vi "CCD_Initialization.vi"(0 "CCD GPIB Address":i16=1 min=1 max=1, 1 "milliseconds to wait":u32=1000, 2 "Setup String":string="LDu,0,256,8;SDu,0,1024,1024;CL4;OMrm;SRon", 3 "error in":errorcluster, 4 "Starting Action":T1(ring)=enum."Init GPIB") -> (5 "Setup String sent":string="ldu,0,256,16;sdu,0,1024,1024;cl0;omrm;sron", 6 "Poll Byte":i16, 7 "Poll Status":bool[](array[boolean]), 8 "Error (0=No Error)":i16=-1, 9 "error out":errorcluster)   [LabVIEW 2020]
doc: "Resets the CCD camera controller and initializes it with Setup String. The default Setup String is \"ldb,1,16,u,0,225,25,b,1,15;sdu,0,1024,1024;cl0;omrm;sron\". \nError, if no -1, is set as 0 if a serial poll detects an error (bit 15 in status bit set)\n\nSet the CCD Setup String Global variable after the command is complete."
uses:
  Globals and TypeDefs/Type Definitions.llb/3 way Status.ctl
  Globals and TypeDefs/Error Categories.ctt
  Globals and TypeDefs/gStatus.vi
  Globals and TypeDefs/gDetector.vi
panel:
  in  "Case Constant\n(See Context Help)":bool=TRUE
  out "Current Action":T1(ring)=enum."Init GPIB"
  in  "milliseconds to wait in begin":u32=1000
  out "Poll Status 2":bool[](array[boolean])
  out "SRQWait":errorcluster
  out "SRQ Poll":bool[](array[boolean])
  out "SRQ":bool
  out "SetupTime (ms)":u32=3
  out "Poll StatusNo":u16
  out "GPIB Error":u16
  # "Status Byte:\n[0]: Dev.Clear State  \n[1]: Dev.Trig.State    \n[2]: Listener Active   \n[3]: Talker Active      \n[4]: Attn. Asserted    \n[5]: CIC                      \n[6]: Remote State       \n[7]: Lockout State      \n[8]: Oper.Complete\n[9]:   ---\n[10]: ---\n[11]: ---\n[12]: SRQ det.whl CIC\n[13]: EOI or EOS det.\n[14]: Timeout\n[15]: Error detected"
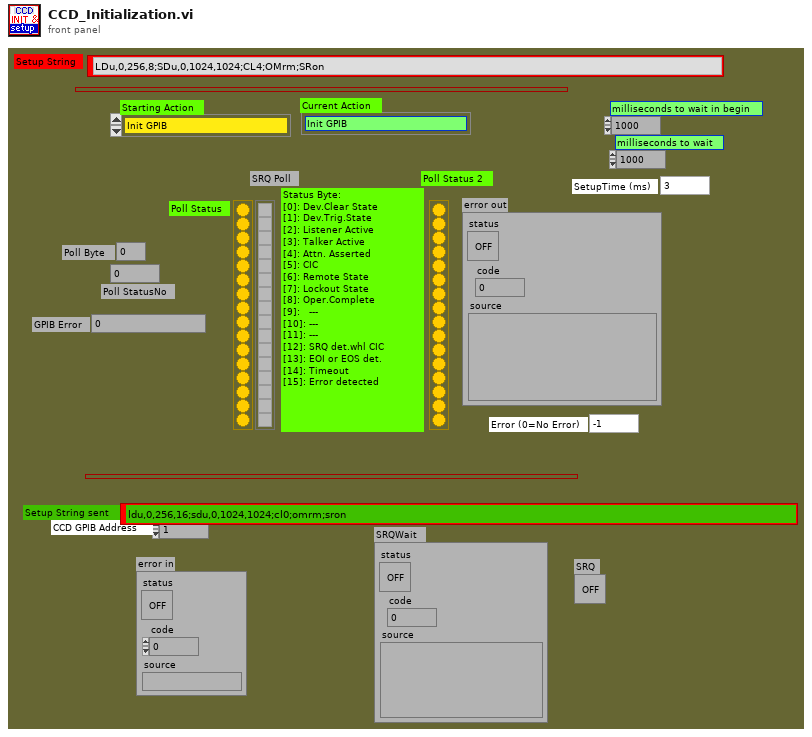
[diagram p1: front panel]
types:
  T1 = enum16{"--Quit--", "Init GPIB", "Poll GPIB", "Wait for SRQ", "Clear CCD Parameters", "New CCD Parameters", "Check CCD Command Error"}
  T2 = enum8{"Initialization Error", "Command Error", "Parameter Error", "Overflow Error", "Time-out Error", "Misc Error", "User cancel"}
  T3 = typedef "Error Categories.ctt" = enum8{"General", "CCD-256x1024", "CCD-1340x400", "InGaAs PDA", "McPherson 2075", "Magnetic Field", "Temperature Control", "Other"}
  T4 = enum16{"Poll CCD GPIB Status", "Check CCD Command Error", "CheckSRQ-Poll"}
  T5 = typedef "3 way Status.ctl" = u8
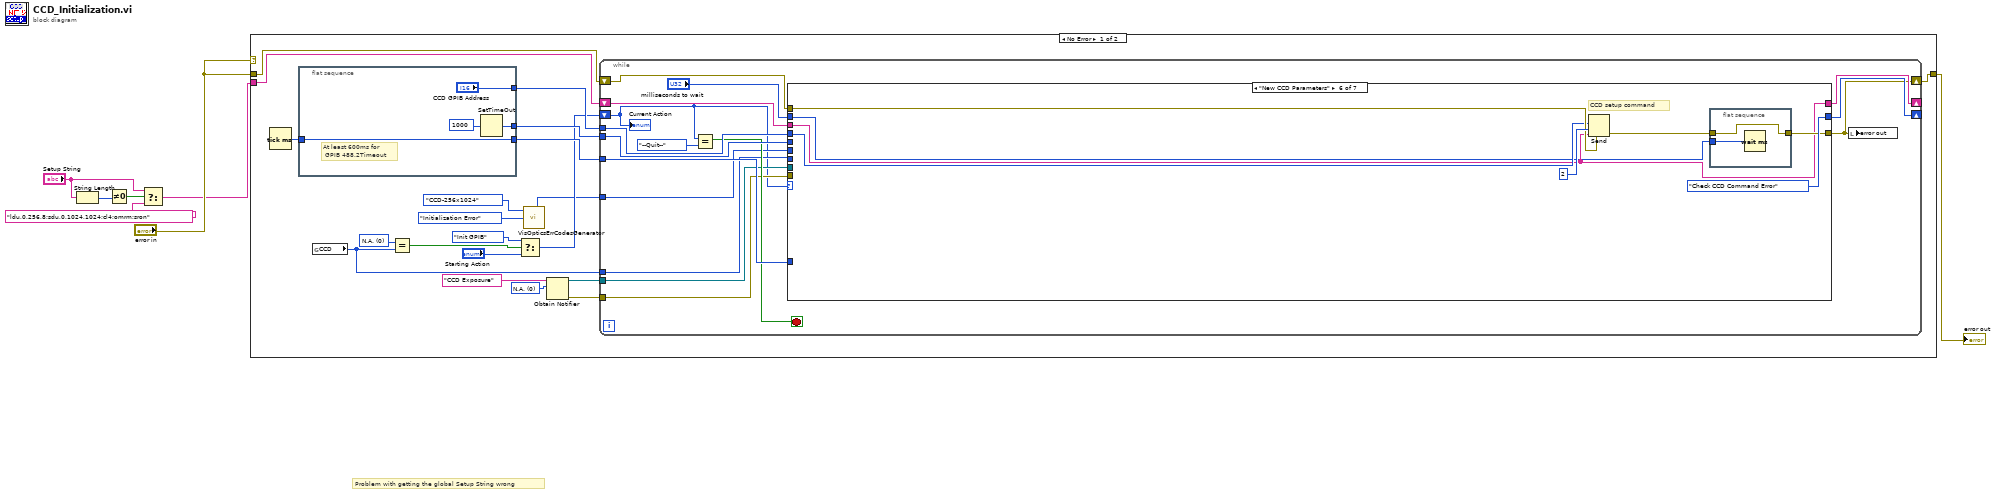
[diagram p0: block diagram]
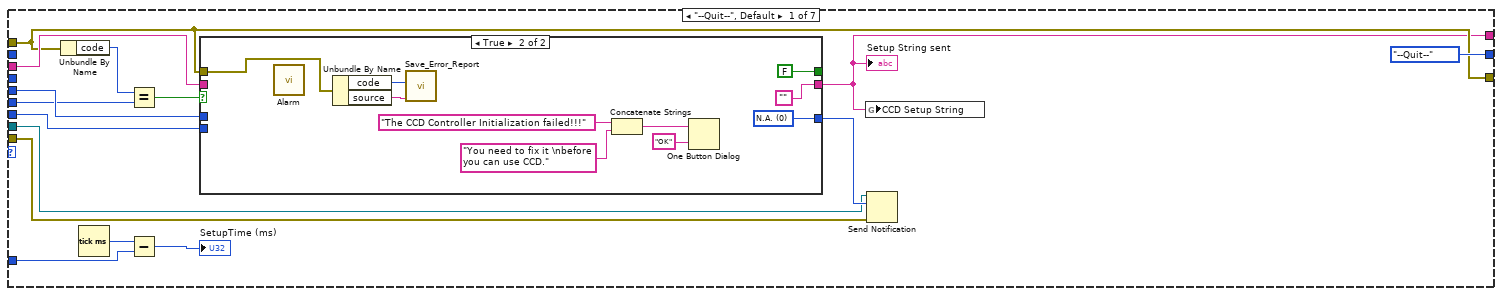
[diagram p2: hidden frame]
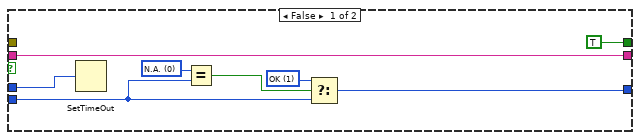
[diagram p3: hidden frame]
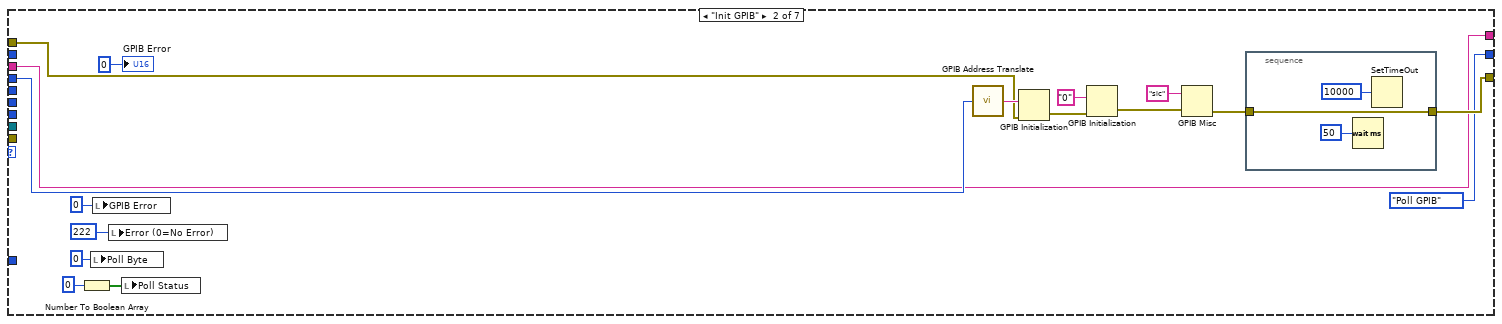
[diagram p4: hidden frame]
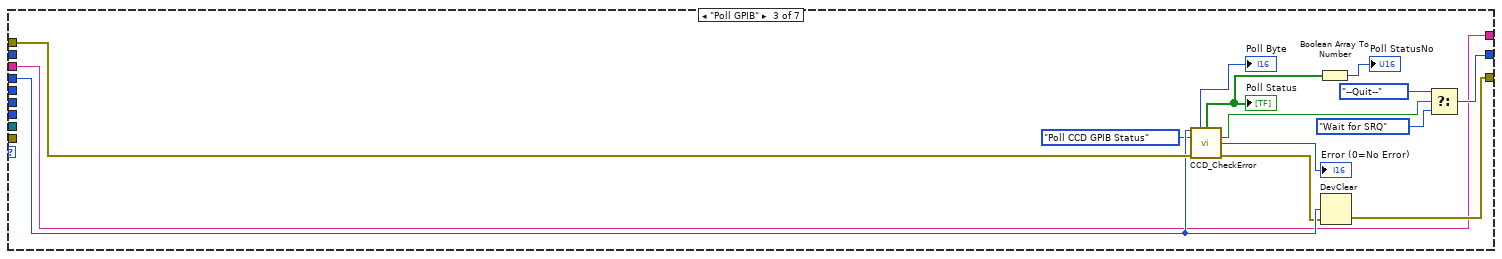
[diagram p5: hidden frame]
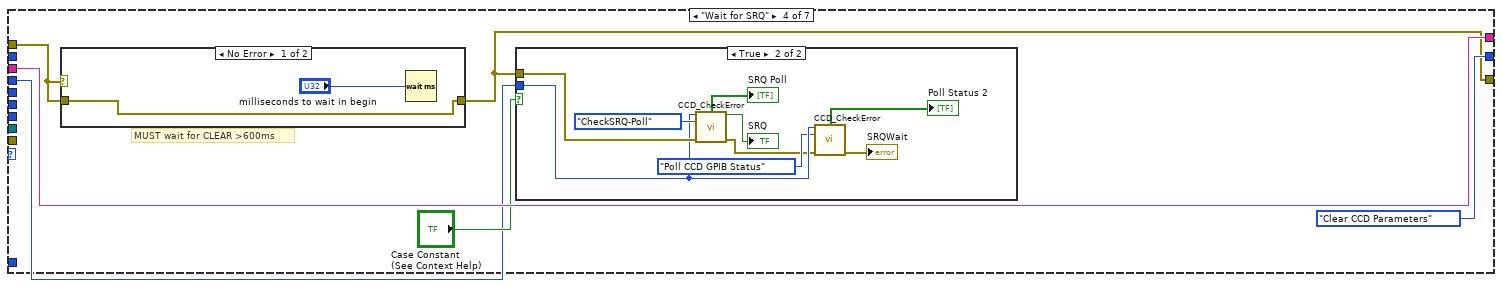
[diagram p6: hidden frame]
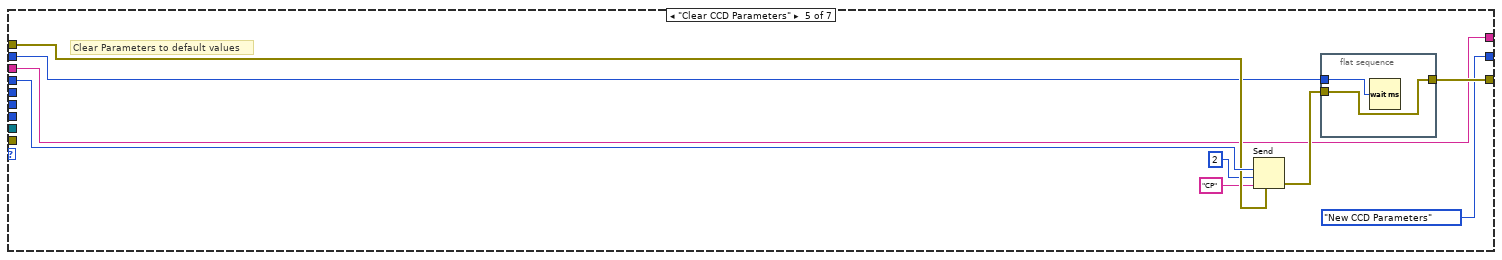
[diagram p9: hidden frame]
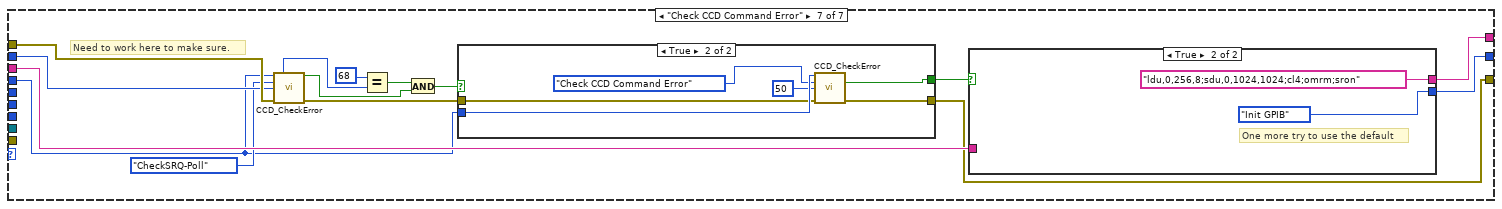
[diagram p10: hidden frame]
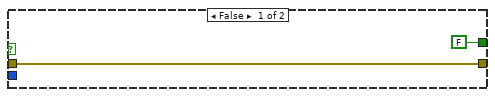
[diagram p11: hidden frame]
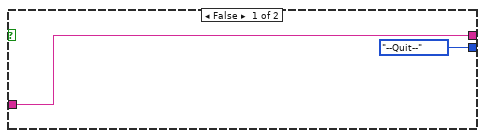
[diagram p12: hidden frame]
diagram:
  # "Problem with getting the global Setup String wrong"
  n1 = String Length(string="Setup String") -> (length=w5:i32)
  n2 = Not Equal To 0?(x=w5) -> (x != 0?=w3:bool)
  n3 = Select(t="Setup String", s=w3, f="ldu,0,256,8;sdu,0,1024,1024;cl4;omrm;sron") -> (s? t:f=w1:string)
  n4 = case shown="No Error" "error in" {
    tunnel: "error in" -> [w27 w181]
    tunnel: [w25 w181] -> w7
    tunnel: w1 -> [w8 _]
    frame No Error {
      w14 = T5 0 items=["N.A.", "OK", "Busy", "Done"] ("Saving")
      w17 = T5 0 items=["N.A.", "OK", "Busy", "Done"] ("y")
      n5 = Tick Count (ms)() -> (millisecond timer value=w23:u32)
      n6 = flat-sequence {
        tunnel: ["CCD GPIB Address"] -> w26
        tunnel: [w30] -> w24
        tunnel: w23 -> [w28]
        tunnel: [w28] -> w22
        frame #0 {
          # "At least 600ms for \n GPIB 488.2Timeout"
          n7 = SetTimeOut(1:1000 ("new timeout (10000)")) -> (0:w30:i32)
        }
      }
      n8 = global read "gStatus.vi" "CCD"() -> (w16:T5)
      n9 = Equal?(x=w17, y=w16) -> (x = y?=w21:bool)
      n10 = Select(t=T1."Init GPIB", s=w21, f="Starting Action") -> (s? t:f=w19:T1)
      n11 = call "VisOpticsErrCodesGenerator.vi"("NHMFL Visible Optics Error Type"=T2."Initialization Error", "NHMFL Visible Optics Error Categories"=Error_Categories.ctt."CCD-256x1024") -> ("User-defined Error Code"=w9:i32)  [unwired: 1 in, 5 out]
      n12 = Obtain Notifier(name (unnamed)="CCD Exposure", notification data type=w14) -> (notifier out=w13:refnum<notifier>, error out=w12:errorcluster)  [unwired: 2 in, 1 out]
      n13 = while {
        shift-right: [w32] -> w25
        shift-left: w27 -> [w47]
        tunnel: w22 -> [w45]
        tunnel: w26 -> [w46]
        tunnel: w24 -> [w44]
        shift-right: [w41] -> _
        shift-left: w19 -> [w33]
        shift-right: [w39] -> _
        shift-left: w8 -> [w40]
        tunnel: w13 -> [w38]
        tunnel: w12 -> [w37]
        tunnel: w16 -> [w34]
        tunnel: w9 -> [w36]
        stop <- w43 stop-if-true
        n14 = Equal?(x=w33, y=T1."--Quit--" ("Starting Action")) -> (x = y?=w43:bool)
        n15 = case shown="\"New CCD Parameters\"" w33 {
          tunnel: w47 -> [w50 w86 w110 w120 w140 w150 w165]
          tunnel: w46 -> [_ w85 w109 w115 w141 w148 w162]
          tunnel: [w50 w83 w103 w117 w137 w146 w154] -> w32
          tunnel: w40 -> [w57 w81 w101 w118 w135 w145 w166]
          tunnel: w45 -> [w62 _ _ _ _ _ _]
          tunnel: w44 -> [w59 _ _ _ _ _ _]
          tunnel: [T1."--Quit--" ("Starting Action") T1."Poll GPIB" ("Starting Action") w114 T1."Clear CCD Parameters" ("Starting Action") T1."New CCD Parameters" ("Starting Action") T1."Check CCD Command Error" ("Starting Action") w168] -> w41
          tunnel: [w49 w81 w101 w118 w135 w145 w167] -> w39
          tunnel: w38 -> [w55 _ _ _ _ _ _]
          tunnel: w37 -> [w54 _ _ _ _ _ _]
          tunnel: w36 -> [w52 _ _ _ _ _ _]
          tunnel: "milliseconds to wait" -> [_ _ _ _ w134 w144 w164]
          tunnel: w34 -> [w48 _ _ _ _ _ _]
          frame "--Quit--", Default {
            n16 = Unbundle By Name(w50) -> ("code"=w53:i32)
            n17 = Tick Count (ms)() -> (millisecond timer value=w61:u32)
            n18 = Equal?(x=w53, y=w52) -> (x = y?=w51:bool)
            n19 = Subtract(x=w61, y=w62) -> (x-y=→"SetupTime (ms)":u32)
            n20 = case shown="True" w51 {
              tunnel: [w68 ""] -> w49
              tunnel: w57 -> [w68 _]
              tunnel: w59 -> [w70 _]
              tunnel: [w63 w73] -> w56
              tunnel: [TRUE ("CCD OK?") FALSE ("CCD OK?")] -> _
              tunnel: w50 -> [_ w71]
              tunnel: w48 -> [w64 _]
              frame False {
                w65 = T5 1 items=["N.A.", "OK", "Busy", "Done"] ("Exposure")
                w67 = T5 0 items=["N.A.", "OK", "Busy", "Done"] ("x")
                n21 = SetTimeOut(1:w70) -> ()  [unwired: 1 out]
                n22 = Equal?(x=w67, y=w64) -> (x = y?=w66:bool)
                n23 = Select(t=w65, s=w66, f=w64) -> (s? t:f=w63:T5)
              }
              frame True {
                w73 = T5 0 items=["N.A.", "OK", "Busy", "Done"] ("Exposure")
                n24 = call "Alarm.vi"() -> ()  [unwired: 4 in]
                n25 = Unbundle By Name(w71) -> ("code"=w76:i32, "source"=w75:string)
                n26 = call "Save_Error_Report.VI"("Error Message"=w75, "Error Code (0: No Error)"=w76) -> ()  [unwired: 4 in, 1 out]
                n27 = Concatenate Strings("The CCD Controller Initialization failed!!!" ("message"), "You need to fix it \nbefore you can use CCD." ("message")) -> (w77:string)
                n28 = One Button Dialog(message=w77, button name ("OK")="OK") -> ()  [unwired: 1 out]
              }
            }
            "Setup String sent" <- w49
            n29 = global write "gDetector.vi" "CCD Setup String"(w49) -> ()
            n30 = Send Notification(notification=w56, notifier=w55, error in (no error)=w54) -> ()  [unwired: 2 out]
          }
          frame "Init GPIB" {
            n31 = Number To Boolean Array(number=u16 0) -> (Boolean array=w95:bool[])
            n32 = local write "Poll Byte"(i16 0) -> ()
            n33 = local write "GPIB Error"(u16 0) -> ()
            n34 = local write "Error (0=No Error)"(i16 222) -> ()
            n35 = local write "Poll Status"(w95) -> ()
            n36 = call "GPIB Address Translate.vi"("GPIB Address"=w85) -> ("GPIB Address String"=w91:string)
            n37 = GPIB Initialization(4:w86, 6:w91) -> (0:w88:errorcluster)  [unwired: 5 in]
            n38 = GPIB Initialization(4:w88, 6:"0" ("address string")) -> (0:w89:errorcluster)  [unwired: 5 in]
            n39 = GPIB Misc(0:"sic", 1:w89) -> (4:w84:errorcluster)  [unwired: 2 out]
            n40 = stacked-sequence {
              tunnel: w84 -> [w100]
              tunnel: [w100] -> w83
              frame #0 {
                n41 = Wait (ms)(milliseconds to wait=u32 50) -> ()  [unwired: 1 out]
                n42 = SetTimeOut(1:10000 ("new timeout (10000)")) -> ()  [unwired: 1 out]
              }
            }
            "GPIB Error" <- u16 0
          }
          frame "Poll GPIB" {
            n43 = call "CCD_CheckError.vi"("CCD GPIB Address"=w109, "Mode"=T4."Poll CCD GPIB Status", "error in"=w110) -> ("Poll Byte"=→"Poll Byte":i16, "Poll Status"=w105:bool[], "CCD Error?"=w113:bool, "Error (0=No Error)"=→"Error (0=No Error)":i16, "error out"=w107:errorcluster)  [unwired: 4 in, 4 out]
            "Poll Status" <- w105
            n44 = Boolean Array To Number(Boolean array=w105) -> (number=→"Poll StatusNo":u32)
            n45 = DevClear(2:w107, 3:w109) -> (0:w103:errorcluster)  [unwired: 1 in, 1 out]
            n46 = Select(t=T1."--Quit--" ("Starting Action"), s=w113, f=T1."Wait for SRQ" ("Starting Action")) -> (s? t:f=w114:T1)
          }
          frame "Wait for SRQ" {
            # "MUST wait for CLEAR >600ms"
            n47 = case shown="No Error" w120 {
              tunnel: w120 -> [w131 w132]
              tunnel: [w131 w132] -> w117
              frame No Error {
                n48 = Wait (ms)(milliseconds to wait="milliseconds to wait in begin") -> ()  [unwired: 1 out]
              }
              frame Error {
              }
            }
            n49 = case shown="True" "Case Constant\n(See Context Help)" {
              tunnel: w117 -> [_ w128]
              tunnel: w115 -> [_ w125]
              frame False {
              }
              frame True {
                n50 = call "CCD_CheckError.vi"("CCD GPIB Address"=w125, "Mode"=T4."CheckSRQ-Poll", "error in"=w128) -> ("Poll Status"=→"SRQ Poll":bool[], "SRQ"=→"SRQ":bool, "error out"=w123:errorcluster)  [unwired: 4 in, 6 out]
                n51 = call "CCD_CheckError.vi"("CCD GPIB Address"=w125, "Mode"=T4."Poll CCD GPIB Status", "error in"=w123) -> ("Poll Status"=→"Poll Status 2":bool[], "error out"=→"SRQWait":errorcluster)  [unwired: 4 in, 7 out]
              }
            }
          }
          frame "Clear CCD Parameters" {
            # "Clear Parameters to default values"
            n52 = Send(2:w141, 3:i16 2 ("mode"), 4:w140, 5:"CP") -> (8:w138:errorcluster)  [unwired: 1 in, 2 out]
            n53 = flat-sequence {
              tunnel: w138 -> [w143]
              tunnel: [w143] -> w137
              tunnel: w134 -> [w142]
              frame #0 {
                n54 = Wait (ms)(milliseconds to wait=w142) -> ()  [unwired: 1 out]
              }
            }
          }
          frame "New CCD Parameters" {
            # "CCD setup command"
            n55 = Send(2:w148, 3:i16 2, 4:w150, 5:w145) -> (8:w149:errorcluster)  [unwired: 1 in, 2 out]
            n56 = flat-sequence {
              tunnel: w149 -> [w153]
              tunnel: [w153] -> w146
              tunnel: w144 -> [w152]
              frame #0 {
                n57 = Wait (ms)(milliseconds to wait=w152) -> ()  [unwired: 1 out]
              }
            }
          }
          frame "Check CCD Command Error" {
            # "Need to work here to make sure."
            n58 = call "CCD_CheckError.vi"("CCD GPIB Address"=w162, "Mode"=T4."CheckSRQ-Poll", "milliseconds to wait"=w164, "error in"=w165) -> ("Poll Byte"=w161:i16, "SRQ"=w158:bool, "error out"=w156:errorcluster)  [unwired: 3 in, 6 out]
            n59 = Equal?(x=i16 68, y=w161) -> (x = y?=w159:bool)
            n60 = And(x=w159, y=w158) -> (x .and. y?=w157:bool)
            n61 = case shown="True" w157 {
              tunnel: w162 -> [_ w176]
              tunnel: w156 -> [w169 w174]
              tunnel: [FALSE ("CCD Error?") w173] -> w155
              tunnel: [w169 w172] -> w154
              frame False {
              }
              frame True {
                n62 = call "CCD_CheckError.vi"("CCD GPIB Address"=w176, "Mode"=T4."Check CCD Command Error", "milliseconds to wait"=u32 50, "error in"=w174) -> ("CCD Error?"=w173:bool, "error out"=w172:errorcluster)  [unwired: 3 in, 7 out]
              }
            }
            n63 = case shown="True" w155 {
              tunnel: [T1."--Quit--" ("f") T1."Init GPIB" ("Starting Action")] -> w168
              tunnel: [w177 "ldu,0,256,8;sdu,0,1024,1024;cl4;omrm;sron"] -> w167
              tunnel: w166 -> [w177 _]
              frame False {
              }
              frame True {
                # "One more try to use the default"
              }
            }
          }
        }
        n64 = local write "error out"(w32) -> ()
        "Current Action" <- w33
      }
    }
    frame Error {
    }
  }
  "error out" <- w7
